vi "FGV.vi"(7 "Action":T1, 8 "error in (no error)":errorcluster, 9 "Plugin's IDN":string, 10 "Parent Class":refnum<class "uPluggable.lvclass">, 11 "uPlugin_Handler In":refnum<class "uPlugin_Handler.lvclass">) -> (0 "error out":errorcluster, 1 "Plugin":refnum<class "uPluggable.lvclass">)   [LabVIEW 2021, in "uPlug.lvlib" / "uPlugin_Handler.lvclass"]
uses:
  uPlugin_Handler.lvclass
  TypeDef_FGV Actions.ctl
  uPluggable/uPluggable.lvclass
  uPlugin_Handler.lvclass/uPlugin_Handler.ctl
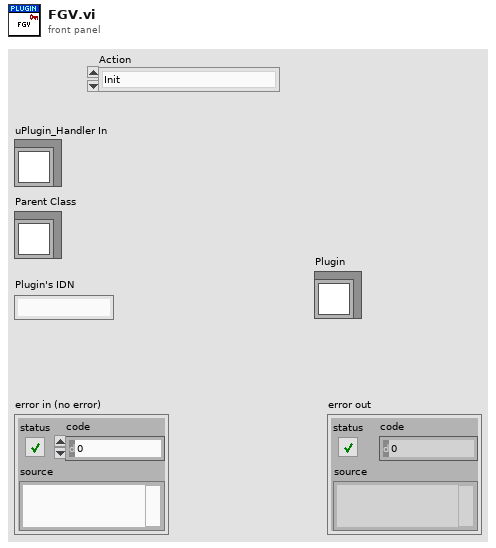
[diagram p1: front panel]
types:
  T1 = typedef "uPlug.lvlib/uPlugin_Handler.lvclass/TypeDef_FGV Actions.ctl" = enum16{"Init", "Load"}
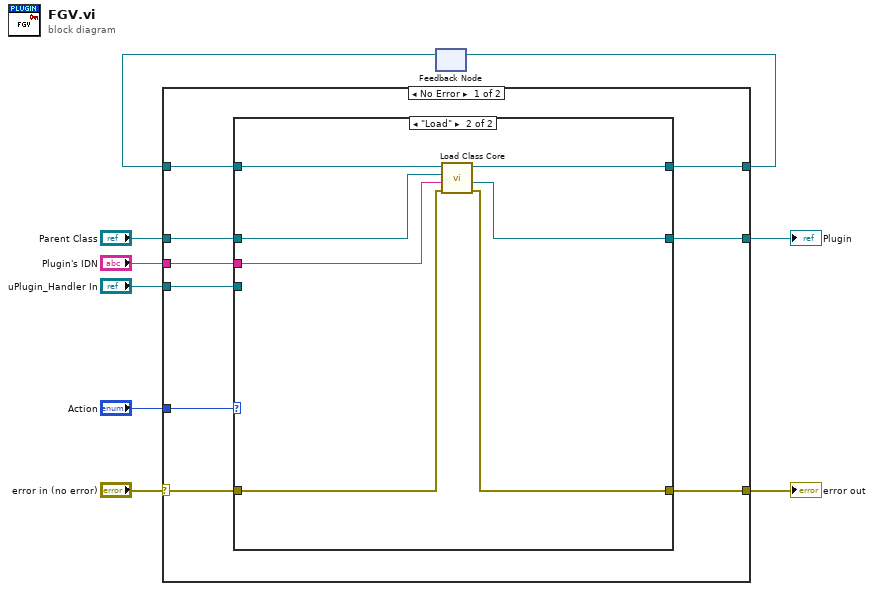
[diagram p0: block diagram]
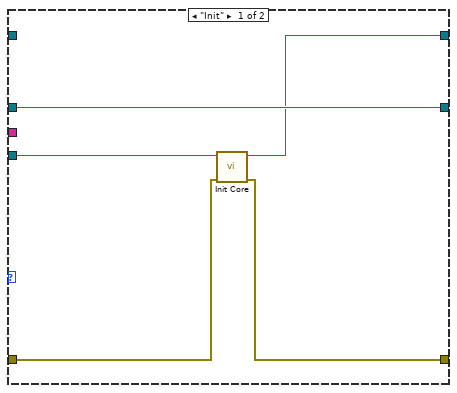
[diagram p2: hidden frame]
diagram:
  n1 = feedback #1() -> (w4:refnum<class "uPlugin_Handler.lvclass">)  [unwired: 1 in]
  n2 = case shown="No Error" "error in (no error)" {
    selector: "error in (no error)" -> [w14 w31]
    tunnel: [w18 w33] -> w5
    tunnel: "uPlugin_Handler In" -> [w17 _]
    tunnel: "Action" -> [w16 _]
    tunnel: [w15 w31] -> w6
    tunnel: w4 -> [w13 w33]
    tunnel: "Plugin's IDN" -> [w12 _]
    tunnel: "Parent Class" -> [w11 w32]
    tunnel: [w10 w32] -> w1
    frame No Error {
      n3 = case shown="\"Load\"" w16 {
        tunnel: w13 -> [_ w29]
        tunnel: [w22 w30] -> w18
        tunnel: w17 -> [w21 _]
        tunnel: [w20 w27] -> w15
        tunnel: w14 -> [w19 w28]
        tunnel: w12 -> [_ w26]
        tunnel: w11 -> [w23 w25]
        tunnel: [w23 w24] -> w10
        frame "Init" {
          n4 = call-dynamic "Init Core.vi"("error in (no error)"=w19, "uPlugin_Handler in"=w21) -> ("error out"=w20:errorcluster, "uPlugin_Handler"=w22:refnum<class "uPlugin_Handler.lvclass">)  [unwired: 8 in]
        }
        frame "Load" {
          n5 = call-dynamic "Load Class Core.vi"("error in (no error)"=w28, "Plugin's IDN"=w26, "Parent Class"=w25, "uPlugin_Handler in"=w29) -> ("error out"=w27:errorcluster, "Plugin"=w24:refnum<class "uPluggable.lvclass">, "uPlugin_Handler out"=w30:refnum<class "uPlugin_Handler.lvclass">)  [unwired: 5 in]
        }
      }
    }
    frame Error {
    }
  }
  "error out" <- w6
  "Plugin" <- w1
  n6 = feedback-in #1(w5) -> ()
